vi "Check If File Already In Database.vi"(8 "error in (no error)":errorcluster, 11 "Path":path) -> (0 "error out":errorcluster, 3 "Already in Database?":bool)   [LabVIEW 2018, in "Database.lvlib"]
uses:
  Database.lvlib
panel:
  out "Output Data [Debug]":string[][](array[string])
  out "Query [debug]":string
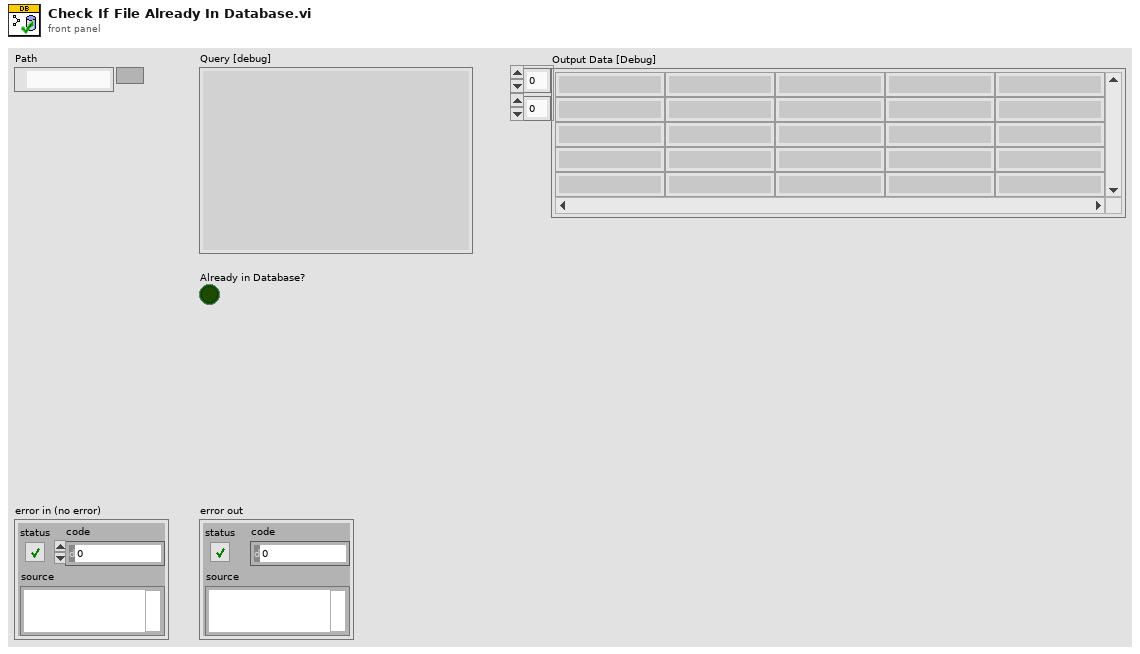
[diagram p1: front panel]
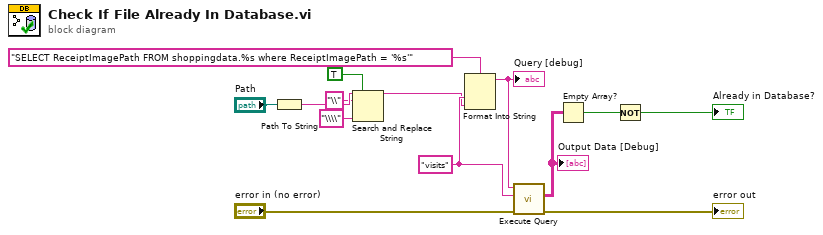
[diagram p0: block diagram]
diagram:
  w11 = "visits" ("input 1")
  n1 = Path To String(path="Path") -> (string=w4:string)
  n2 = Search and Replace String(replace all?=TRUE ("replace all? (F)"), input string=w4, search string="\\", replace string="\\\\" ("replace string (\"\")")) -> (result string=w3:string)  [unwired: 4 in, 3 out]
  n3 = Format Into String(format string="SELECT ReceiptImagePath FROM shoppingdata.%s where ReceiptImagePath = '%s'", w11, w3) -> (resulting string=w7:string)  [unwired: 2 in, 1 out]
  "Query [debug]" <- w7
  n4 = call "Execute Query.vi"("Error In"="error in (no error)", "Table"=w11, "Query"=w7) -> ("Error Out"=→"error out":errorcluster, "Output Data"=w12:string[][])  [unwired: 6 in, 1 out]
  "Output Data [Debug]" <- w12
  n5 = Empty Array?(array=w12) -> (empty?=w13:bool)
  n6 = Not(x=w13) -> (.not. x?=→"Already in Database?":bool)
